vi "Query DUT SIM Slot IMS Supported.vi"(8 "error in (no error)":errorcluster, 9 "SIM Slot (1)":i32=1, 10 "DUT (\"DUT1\")":string="DUT1", 11 "VISA resource name":refnum<visa-resource-name>) -> (0 "error out":errorcluster, 2 "IMS Supported":bool, 3 "VISA resource name out":refnum<visa-resource-name>)   [LabVIEW 2015, in "Rohde&Schwarz CMXP Base.lvlib"]
doc: "Queries whether the inactive DUT supports IP multimedia subsystem (IMS) services.\n\nAttribute:\nRSCMXPBASE_ATTR_SELECT_DUT_SIM_SLOT\n\nRemote-control command:\n[CONFigure:]DUT:PROFile:SIMSlot<no>:CAPability:IMS?"
uses:
  <instrlib>/Rohde&Schwarz CMXP Base/Rohde&Schwarz CMXP Base.lvlib
  <instrlib>/Rohde&Schwarz CMXP Base/Private/rsidr_core.llb/rsidr_core.lvlib
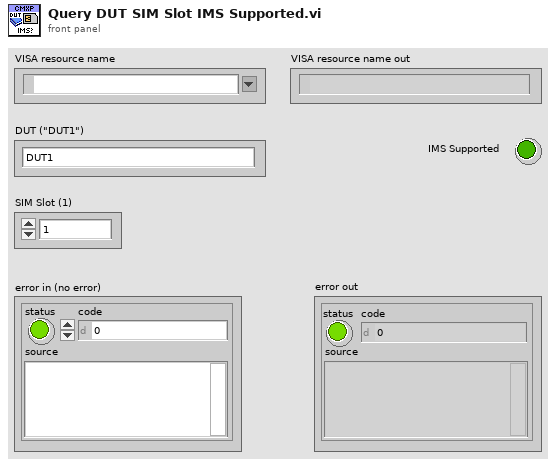
[diagram p1: front panel]
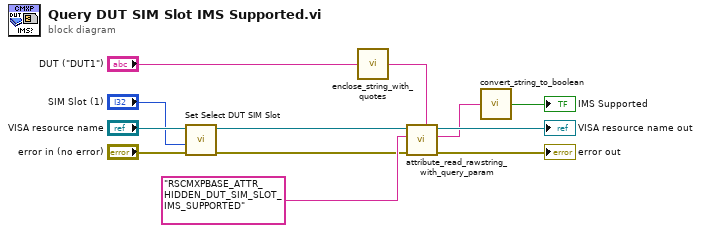
[diagram p0: block diagram]
diagram:
  n1 = call "Set Select DUT SIM Slot"("error in (no error)"="error in (no error)", "Select DUT SIM Slot (0)"="SIM Slot (1)", "instrument handle"="VISA resource name") -> ("error out"=w4:errorcluster, "instrument handle out"=w7:refnum<visa-resource-name>)  [unwired: 7 in]
  n2 = call <instrlib>:"enclose_string_with_quotes.vi"("String to enclose"="DUT (\"DUT1\")") -> ("String out"=w1:string)  [unwired: 4 in]
  n3 = call <instrlib>:"attribute_read_rawstring_with_query_param.vi"("Query Parameter (None)"=w1, "error in"=w4, "Attribute ID"="RSCMXPBASE_ATTR_HIDDEN_DUT_SIM_SLOT_IMS_SUPPORTED", "VISA resource name"=w7) -> ("error out"=→"error out":errorcluster, "RawString out"=w5:string, "VISA resource name out"=→"VISA resource name out":refnum<visa-resource-name>)  [unwired: 5 in]
  n4 = call <instrlib>:"convert_string_to_boolean.vi"("String in"=w5) -> ("boolean value out"=→"IMS Supported":bool)  [unwired: 4 in]
